vi "ScriptFunctions.vi"   [LabVIEW 2017]
uses:
  <vilib>/Utility/traverseref.llb/TRef TravTarget.ctl
  <vilib>/Utility/traverseref.llb/VI Scripting - Traverse.lvlib
types:
  T1 = enum32{"invalid VI type", "Standard VI", "Control VI", "Global VI", "Polymorphic VI", "Configuration VI", "SubSystem", "Facade VI", "Method VI", "Statechart Diagram VI"}
  T2 = cluster{"VIPath":path, "Menu Name":string, "Selector Name":string}
  T3 = typedef "TRef TravTarget.ctl" = enum16{"FP", "BD", "Other"}
  T4 = typedef "imagedata.ctl" = cluster{"image type":i32, "image depth":i32, "image":u8[], "mask":u8[], "colors":u32[], "Rectangle":cluster{"left":i16, "top":i16, "right":i16, "bottom":i16}}
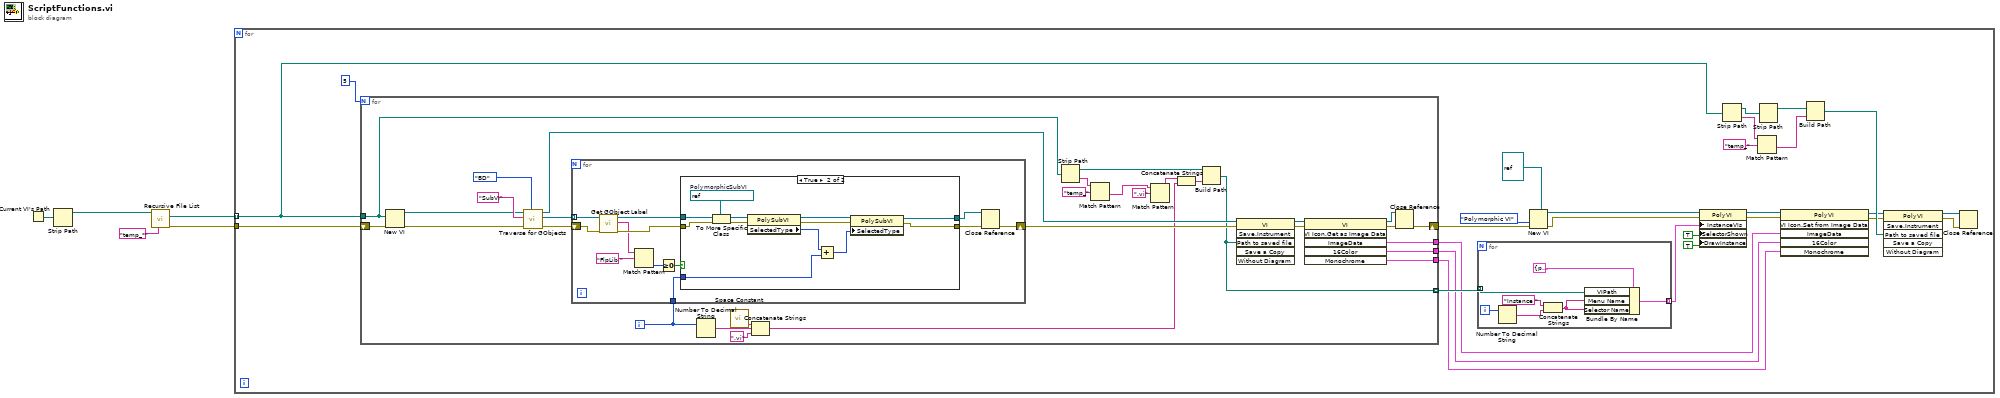
[diagram p0: block diagram]
diagram:
  n1 = Current VI's Path() -> (path=w2:path)
  n2 = Strip Path(path=w2) -> (stripped path=w1:path)  [unwired: 1 out]
  n3 = call <vilib>:"Recursive File List.vi"("pattern"="temp_*", "Folder Path"=w1) -> ("error out"=w3:errorcluster, "All Files in Dir"=w4:path[])  [unwired: 5 in, 3 out]
  n4 = for {
    tunnel: w4 -> [w19] mode=indexing
    tunnel: w3 -> [w18]
    n5 = for {
      N: 5 -> [_]
      tunnel: w19 -> [w64]
      shift-right: [w55] -> w31
      shift-left: w18 -> [w62]
      tunnel: [w56] -> w24 mode=indexing
      tunnel: [w42] -> w10
      tunnel: [w41] -> w9
      tunnel: [w40] -> w6
      i -> [w54]
      n6 = New VI(8:w62, 10:w64) -> (0:w47:errorcluster, 3:w48:refnum<vi>)  [unwired: 5 in]
      n7 = call <vilib>:"Traverse for GObjects.vi"("Traverse Target"=TRef_TravTarget."BD", "error in (no error)"=w47, "Class Name"="SubVI", "VI Refnum"=w48) -> ("error out"=w69:errorcluster, "References"=w68:refnum<vi>[], "dup VI Refnum"=w66:refnum<vi>)  [unwired: 4 in, 1 out]
      n8 = for {
        tunnel: w68 -> [w81] mode=indexing
        shift-right: [w73] -> w65
        shift-left: w69 -> [w82]
        tunnel: w54 -> [w71]
        n9 = call <vilib>:"Get GObject Label.vi"("error in (no error)"=w82, "GObject"=w81) -> ("error out"=w76:errorcluster, "Object Label"=w75:string, "dup GObject"=w77:refnum<vi>)  [unwired: 5 in, 2 out]
        n10 = Match Pattern(string=w75, regular expression="FlpLib ") -> (offset past match=w79:i32)  [unwired: 1 in, 3 out]
        n11 = Greater Or Equal To 0?(x=w79) -> (x >= 0?=w78:bool)
        n12 = case shown="True" w78 {
          tunnel: w77 -> [w83 w96]
          tunnel: w76 -> [w84 w94]
          tunnel: [w84 w85] -> w74
          tunnel: [w83 w87] -> w72
          tunnel: w71 -> [_ w86]
          frame False {
          }
          frame True {
            w95 = refnum<vi> refnum  # PolymorphicSubVI
            n13 = To More Specific Class(target class=w95, reference=w96, error in=w94) -> (specific class reference=w93:refnum<vi>, error out=w92:errorcluster)
            n14 = property class="PolySubVI"(reference=w93, error in=w92) -> (reference out=w91:refnum<vi>, error out=w90:errorcluster, "SelectedType"=w89:i32)
            n15 = Add(x=w89, y=w86) -> (x+y=w88:i32)
            n16 = property class="PolySubVI"(reference=w91, error in=w90, "SelectedType"=w88) -> (reference out=w87:refnum<vi>, error out=w85:errorcluster)
          }
        }
        n17 = Close Reference(reference=w72, error in (no error)=w74) -> (error out=w73:errorcluster)
      }
      n18 = Number To Decimal String(number=w54) -> (decimal integer string=w61:string)  [unwired: 1 in]
      n19 = call <vilib>:"Space Constant.vi"() -> ("String"=w59:string)
      n20 = Concatenate Strings(w59, w61, ".vi" ("string")) -> (w58:string)
      n21 = Strip Path(path=w64) -> (stripped path=w63:path, name=w51:string)
      n22 = Match Pattern(string=w51, regular expression="temp_") -> (after substring=w49:string)  [unwired: 1 in, 3 out]
      n23 = Match Pattern(string=w49, regular expression=".vi") -> (before substring=w52:string)  [unwired: 1 in, 3 out]
      n24 = Concatenate Strings(w52, w58) -> (w57:string)
      n25 = Build Path(base path=w63, name or relative path=w57) -> (appended path=w56:path)
      n26 = invoke class="VI" method="Save.Instrument"(reference=w66, error in=w65, "Path to saved file"=w56) -> (reference out=w45:refnum<vi>, error out=w46:errorcluster)  [unwired: 3 in, 4 out]
      n27 = invoke class="VI" method="VI Icon.Get as Image Data"(reference=w45, error in=w46) -> (reference out=w43:refnum<vi>, error out=w44:errorcluster, "ImageData"=w42:T4, "16Color"=w41:T4, "Monochrome"=w40:T4)  [unwired: 4 in, 1 out]
      n28 = Close Reference(reference=w43, error in (no error)=w44) -> (error out=w55:errorcluster)
    }
    n29 = for {
      tunnel: w24 -> [w38] mode=indexing
      tunnel: [w33] -> w23 mode=indexing
      i -> [w37]
      n30 = Number To Decimal String(number=w37) -> (decimal integer string=w35:string)  [unwired: 1 in]
      n31 = Concatenate Strings("Instance ", w35) -> (w34:string)
      n32 = Bundle By Name(cluster=T2 {"VIPath"=path "", "Menu Name"="", "Selector Name"=""}, "VIPath"=w38, "Menu Name"=w34, "Selector Name"=w34) -> (w33:T2)
    }
    n33 = New VI(5:refnum<vi> refnum ("type specifier VI Refnum (for type only)"), 8:w31, 9:T1."Polymorphic VI" ("vi type (standard vi)")) -> (0:w22:errorcluster, 3:w25:refnum<vi>)  [unwired: 4 in]
    n34 = property class="PolyVI"(reference=w25, error in=w22, "InstanceVIs"=w23, "SelectorShown"=TRUE ("Show Selector By Default"), "DrawInstance"=TRUE ("Draw Instance Icon")) -> (reference out=w12:refnum<vi>, error out=w11:errorcluster)
    n35 = Strip Path(path=w19) -> (stripped path=w17:path, name=w16:string)
    n36 = Match Pattern(string=w16, regular expression="temp_") -> (after substring=w13:string)  [unwired: 1 in, 3 out]
    n37 = Strip Path(path=w17) -> (stripped path=w14:path)  [unwired: 1 out]
    n38 = invoke class="PolyVI" method="VI Icon.Set from Image Data"(reference=w12, error in=w11, "ImageData"=w10, "16Color"=w9, "Monochrome"=w6) -> (reference out=w8:refnum<vi>, error out=w7:errorcluster)  [unwired: 1 in, 4 out]
    n39 = Build Path(base path=w14, name or relative path=w13) -> (appended path=w27:path)
    n40 = invoke class="PolyVI" method="Save.Instrument"(reference=w8, error in=w7, "Path to saved file"=w27) -> (reference out=w29:refnum<vi>, error out=w28:errorcluster)  [unwired: 3 in, 4 out]
    n41 = Close Reference(reference=w29, error in (no error)=w28) -> ()  [unwired: 1 out]
  }
